vi "SetCursorPos(ObjectName)Panel.vi"(7 "vi reference":refnum<vi>, 8 "error in":errorcluster, 9 "Relative x,y":T1, 10 "Object Name":string, 11 "owner refnum":refnum<vi>) -> (0 "Error out":errorcluster, 2 "Sucess?":i32, 3 "GObj Refnum Out":refnum<vi>)   [LabVIEW 2013]
uses:
  <vilib>/Utility/miscctls.llb/LVPositionTypeDef.ctl
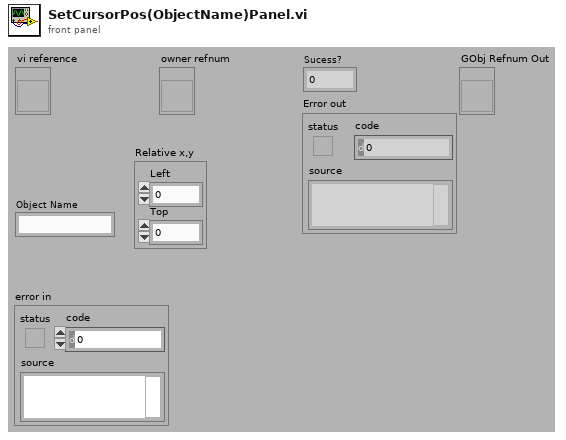
[diagram p1: front panel]
types:
  T1 = typedef "LVPositionTypeDef.ctl" = cluster{"Left":i32, "Top":i32}
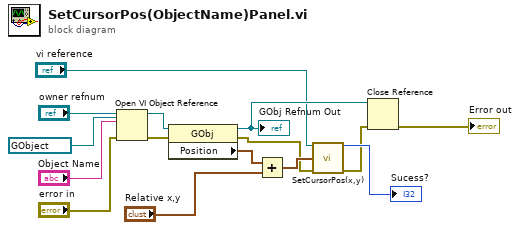
[diagram p0: block diagram]
diagram:
  n1 = Open VI Object Reference(7:refnum<vi> refnum ("GObj Refnum"), 8:"error in", 10:"Object Name", 11:"owner refnum") -> (0:w13:errorcluster, 3:w14:refnum<vi>)
  n2 = property class="GObj"(reference=w14, error in=w13) -> (reference out=w9:refnum<vi>, error out=w2:errorcluster, "Position"=w8:T1)
  "GObj Refnum Out" <- w9
  n3 = Add(x=w8, y="Relative x,y") -> (x+y=w6:T1)
  n4 = call "SetCursorPos(x,y).vi"("vi reference"="vi reference", "(X,Y)"=w6, "Error in"=w2) -> ("Sucess?"=→"Sucess?":i32, "Error out"=w10:errorcluster)  [unwired: 1 in, 10 out]
  n5 = Close Reference(reference=w9, error in (no error)=w10) -> (error out=→"Error out":errorcluster)
